vi "Controller - State Change.vi"(8 "error in (no error)":errorcluster, 11 "View Model":T1) -> (0 "error out":errorcluster, 3 "View Model":T1)   [LabVIEW 2017]
doc: "Processing exit from current Elevator state and\nset up next state as current for next iteration"
uses:
  View Model/Controls/View Model.ctl
  View Model/Controls/Shared Model.ctl
  Error/Controls/Error Model.ctl
  Error/Controls/Error Event.ctl
  Error/Controls/Error Type.ctl
  Configuration/Controls/Config DB Model.ctl
  Configuration/Controls/Config DB Command.ctl
  Configuration/Controls/Config DB Record.ctl
  Controls/Controller Model.ctl
  Controls/Elevator Location.ctl
  Controls/Elevator Direction Event.ctl
  Controls/Elevator Direction.ctl
  Controls/Elevator CMD Event.ctl
  Controls/Elevator Commands.ctl
  Controls/Elevator Overhead.ctl
  Controls/Elevator State.ctl
  Controls/Elevator CMD Timer.ctl
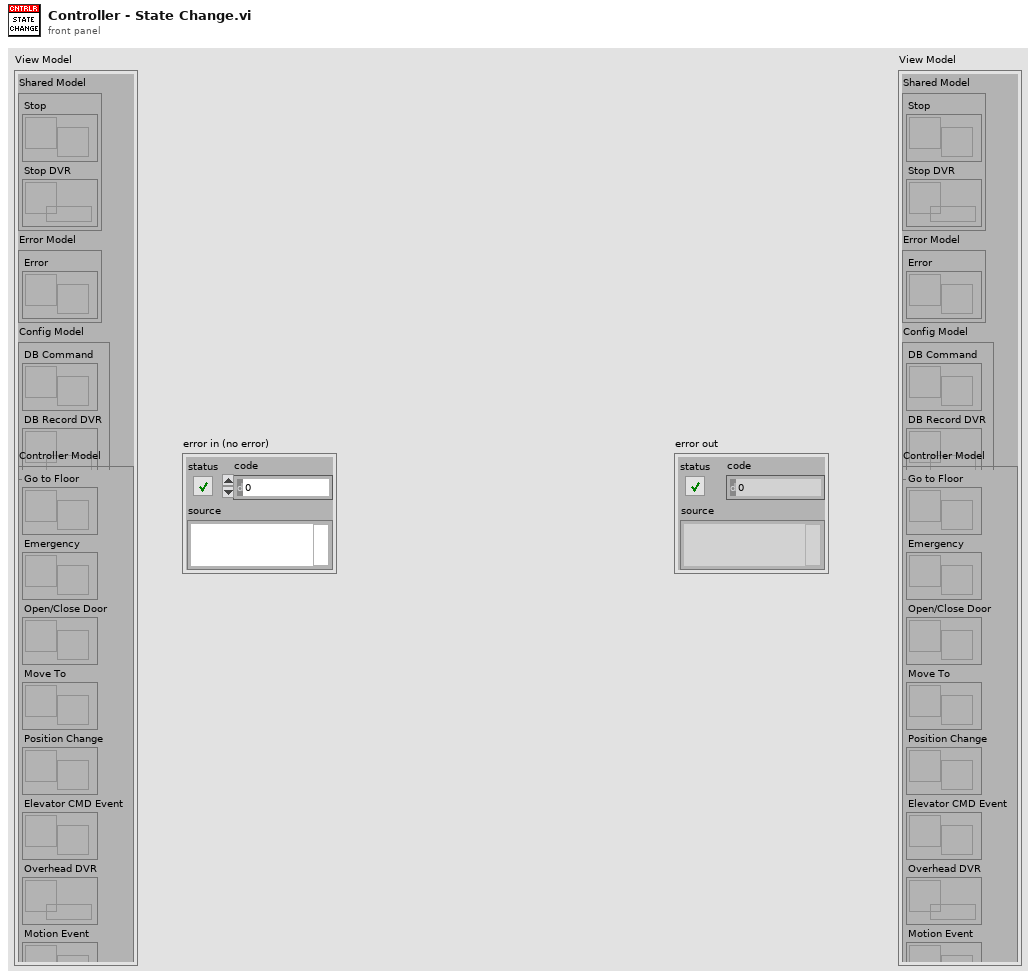
[diagram p1: front panel]
types:
  T1 = typedef "View Model.ctl" = cluster{"Shared Model":T2, "Error Model":T3, "Config Model":T4, "Controller Model":T5}
  T2 = typedef "Shared Model.ctl" = cluster{"Stop":refnum<user-event>, "Stop DVR":refnum<data-value>}
  T3 = typedef "Error Model.ctl" = cluster{"Error":refnum<user-event>}
  T4 = typedef "Config DB Model.ctl" = cluster{"DB Command":refnum<user-event>, "DB Record DVR":refnum<data-value>}
  T5 = typedef "Controller Model.ctl" = cluster{"Go to Floor":refnum<user-event>, "Emergency":refnum<user-event>, "Open/Close Door":refnum<user-event>, "Move To":refnum<user-event>, "Position Change":refnum<user-event>, "Elevator CMD Event":refnum<user-event>, "Overhead DVR":refnum<data-value>, "Motion Event":refnum<user-event>}
  T6 = typedef "Elevator State.ctl" = enum16{"No Request", "Initial", "Wait for 1st Request", "Start and Move", "Analysis", "Continue Travel", "Stop at Floor", "Open/Close Door", "Emergency", "Terminate"}
  T7 = typedef "Elevator CMD Timer.ctl" = enum16{"Start", "Get Time", "Pause", "Unpause"}
  T8 = typedef "Elevator Location.ctl" = enum16{"1st Floor", "2nd Floor", "3rd Floor", "4th Floor"}
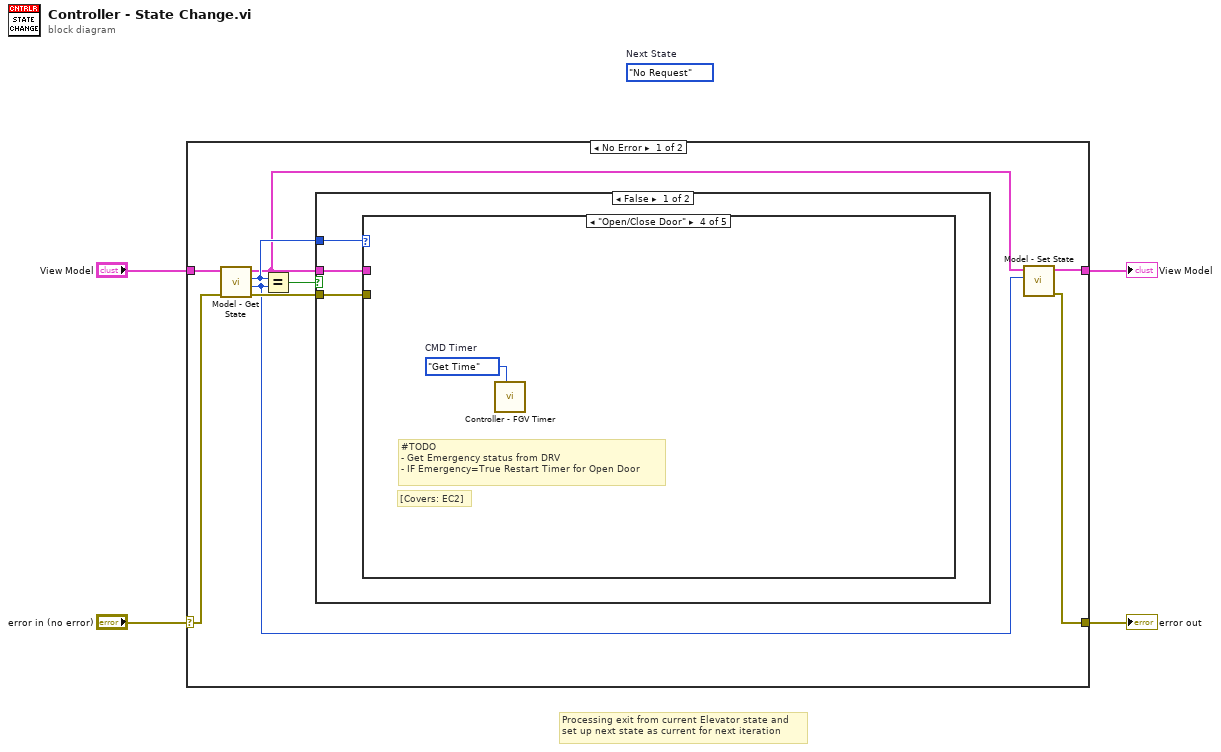
[diagram p0: block diagram]
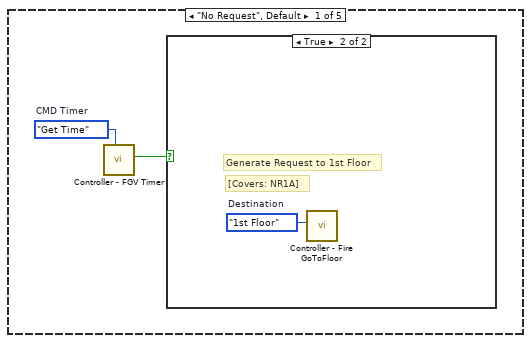
[diagram p2: hidden frame]
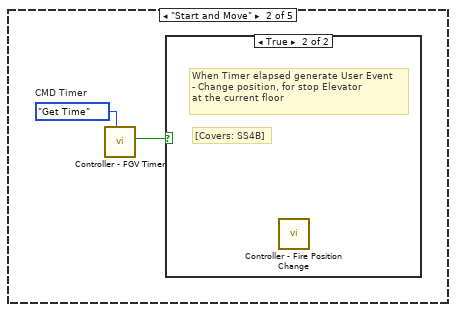
[diagram p4: hidden frame]
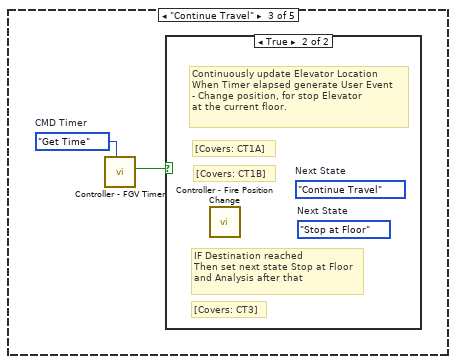
[diagram p6: hidden frame]
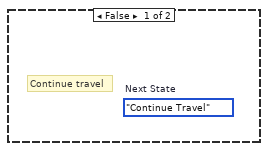
[diagram p7: hidden frame]
diagram:
  (unwired) Elevator_State."No Request"  # Next State
  # "Processing exit from current Elevator state and\nset up next state as current for next iteration"
  n1 = case shown="No Error" "error in (no error)" {
    selector: "error in (no error)" -> [w12 w25]
    tunnel: "View Model" -> [w13 w26]
    tunnel: [w8 w26] -> w2
    tunnel: [w5 w25] -> w1
    frame No Error {
      n2 = call "Model - Get State.vi"("error in (no error)"=w12, "View Model"=w13) -> ("error out"=w10:errorcluster, "Next State"=w6:T6, "Current State"=w9:T6, "View Model"=w7:T1)  [unwired: 6 in]
      n3 = Equal?(x=w9, y=w6) -> (x = y?=w11:bool)
      n4 = case shown="False" w11 {
        tunnel: w10 -> [w14 _]
        tunnel: w7 -> [w15 _]
        tunnel: w9 -> [w16 _]
        frame False {
          n5 = case shown="\"Open/Close Door\"" w16 {
            tunnel: w15 -> [_ _ _ _ _]
            tunnel: w14 -> [_ _ _ _ _]
            frame "No Request", Default {
              w18 = Elevator_CMD_Timer."Get Time"  # CMD Timer
              n6 = call "Controller - FGV Timer.vi"("CMD Timer"=w18) -> ("Elapsed?"=w17:bool)  [unwired: 8 in, 2 out]
              n7 = case shown="True" w17 {
                frame False {
                }
                frame True {
                  w19 = Elevator_Location."1st Floor"  # Destination
                  # "[Covers: NR1A]"
                  # "Generate Request to 1st Floor"
                  n8 = call "Controller - Fire GoToFloor.vi"("Destination"=w19) -> ()  [unwired: 9 in, 2 out]
                }
              }
            }
            frame "Start and Move" {
              w21 = Elevator_CMD_Timer."Get Time"  # CMD Timer
              n9 = call "Controller - FGV Timer.vi"("CMD Timer"=w21) -> ("Elapsed?"=w20:bool)  [unwired: 8 in, 2 out]
              n10 = case shown="True" w20 {
                frame False {
                }
                frame True {
                  # "[Covers: SS4B]"
                  # "When Timer elapsed generate User Event\n- Change position, for stop Elevator\nat the current floor"
                  n11 = call "Controller - Fire Position Change.vi"() -> ()  [unwired: 10 in, 2 out]
                }
              }
            }
            frame "Continue Travel" {
              w23 = Elevator_CMD_Timer."Get Time"  # CMD Timer
              n12 = call "Controller - FGV Timer.vi"("CMD Timer"=w23) -> ("Elapsed?"=w22:bool)  [unwired: 8 in, 2 out]
              n13 = case shown="True" w22 {
                frame False {
                  (unwired) Elevator_State."Continue Travel"  # Next State
                  # "Continue travel"
                }
                frame True {
                  (unwired) Elevator_State."Stop at Floor"  # Next State
                  (unwired) Elevator_State."Continue Travel"  # Next State
                  # "[Covers: CT3]"
                  # "IF Destination reached\nThen set next state Stop at Floor\nand Analysis after that"
                  # "[Covers: CT1B]"
                  # "[Covers: CT1A]"
                  # "Continuously update Elevator Location\nWhen Timer elapsed generate User Event\n- Change position, for stop Elevator\nat the current floor."
                  n14 = call "Controller - Fire Position Change.vi"() -> ()  [unwired: 10 in, 2 out]
                }
              }
            }
            frame "Open/Close Door" {
              w24 = Elevator_CMD_Timer."Get Time"  # CMD Timer
              # "[Covers: EC2]"
              # "#TODO\n- Get Emergency status from DRV\n- IF Emergency=True Restart Timer for Open Door"
              n15 = call "Controller - FGV Timer.vi"("CMD Timer"=w24) -> ()  [unwired: 8 in, 3 out]
            }
            frame "Initial" {
            }
          }
        }
        frame True {
        }
      }
      n16 = call "Model - Set State.vi"("Current State"=w6, "View Model"=w7) -> ("error out"=w5:errorcluster, "View Model"=w8:T1)  [unwired: 8 in]
    }
    frame Error {
    }
  }
  "error out" <- w1
  "View Model" <- w2
